vi "status conditions.vi"(8 "error in":errorcluster, 10 "status":T1=enum."Initialize", 11 "Simulation Controls":T2 {"Water Pressure Sensor (%)" scale=0.0..100.0}) -> (0 "error out":errorcluster, 3 "status out":T1)   [LabVIEW 2015]
uses:
  controls/state.ctl
panel:
  # "Rain"
  # "No Rain"
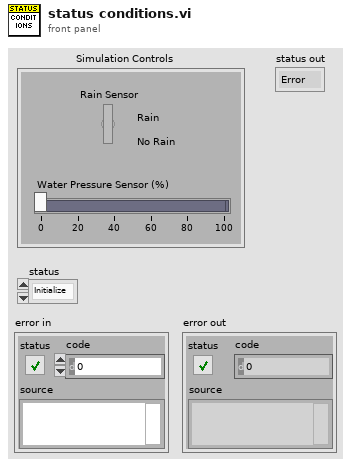
[diagram p1: front panel]
types:
  T1 = typedef "state.ctl" = enum16{"Error", "End", "Start", "Exit", "Setup", "Low pressure", "Rain", "Run", "Idle", "Initialize"}
  T2 = cluster{"Rain Sensor":bool, "Water Pressure Sensor (%)":dbl}
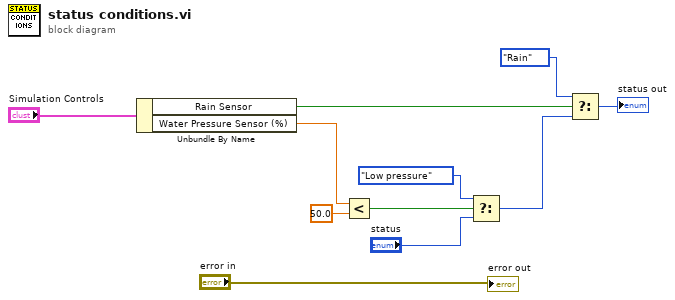
[diagram p0: block diagram]
diagram:
  n1 = Unbundle By Name("Simulation Controls") -> ("Rain Sensor"=w3:bool, "Water Pressure Sensor (%)"=w4:dbl)
  n2 = Less?(x=w4, y=50.0) -> (x < y?=w8:bool)
  n3 = Select(t=state."Low pressure" ("status"), s=w8, f="status") -> (s? t:f=w10:T1)
  n4 = Select(t=state."Rain" ("status"), s=w3, f=w10) -> (s? t:f=→"status out":T1)
  "error out" <- "error in"
